vi "Update Lists From BIMS Server.vi"(4 "error IN":errorcluster, 6 "Site":string, 7 "Lookup Table Name":string) -> (0 "error OUT":errorcluster, 3 "recordset data":string[][](array[string]))   [LabVIEW 2010]
uses:
  <vilib>/addons/database/Connection.llb/DB Tools Open Connec (Path).vi
  <vilib>/addons/database/Connection.llb/Conn Execute.vi
  <vilib>/addons/database/Recordset.llb/Rec Destroy - Connection.vi
  <vilib>/addons/database/NI_Database_API.lvlib
panel:
  out "SP Call":string
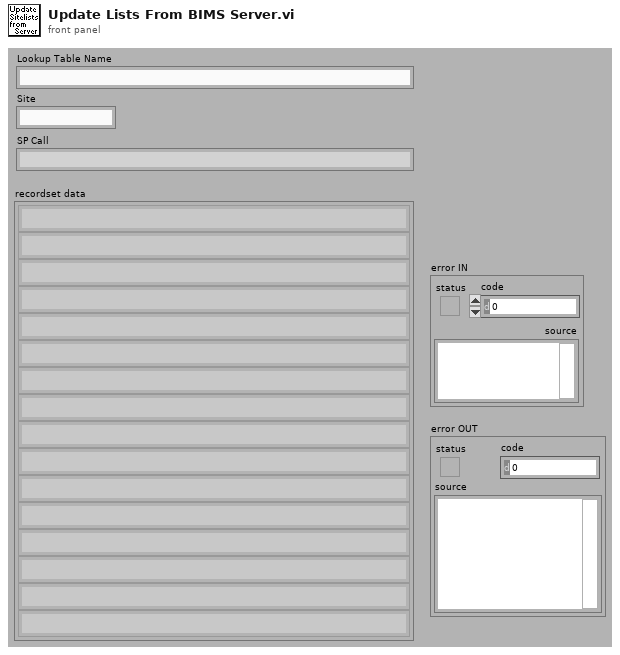
[diagram p1: front panel]
types:
  T1 = typedef "NI_Database_API.lvlib/Conn ObjectReference.ctl" = refnum<k1>
  T2 = typedef "NI_Database_API.lvlib/Rec ObjectReference.ctl" = refnum<k1>
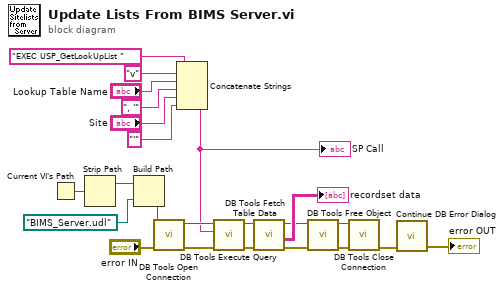
[diagram p0: block diagram]
diagram:
  n1 = Current VI's Path() -> (path=w11:path)
  n2 = Strip Path(path=w11) -> (stripped path=w10:path)  [unwired: 1 out]
  n3 = Build Path(base path=w10, name or relative path=path "BIMS_Server.udl" ("connectString")) -> (appended path=w8:path)
  n4 = call-poly <vilib>:"DB Tools Open Connection.vi"("error in (no error)"="error IN", "connection information"=w8) -> ("error out"=w16:errorcluster, "connection reference"=w14:T1)  [unwired: 3 in, 3 out]
  n5 = Concatenate Strings("EXEC USP_GetLookUpList " ("string"), "v" ("string"), "Lookup Table Name", ", '", "Site", "'") -> (w7:string)
  "SP Call" <- w7
  n6 = call-poly <vilib>:"DB Tools Execute Query.vi"("error in (no error)"=w16, "SQL query"=w7, "connection reference"=w14) -> ("error out"=w17:errorcluster, "recordset reference"=w13:T2)  [unwired: 1 in, 4 out]
  n7 = call <vilib>:"DB Tools Fetch Table Data.vi"("error in (no error)"=w17, "recordset reference"=w13) -> ("error out"=w18:errorcluster, "recordset data"=→"recordset data":string[][], "recordset reference out"=w12:T2)  [unwired: 3 out]
  n8 = call-poly <vilib>:"DB Tools Free Object.vi"("error in (no error)"=w18, "recordset reference"=w12) -> ("error out"=w19:errorcluster, "connection reference"=w15:T1)  [unwired: 8 out]
  n9 = call <vilib>:"DB Tools Close Connection.vi"("error in (no error)"=w19, "connection reference"=w15) -> ("error out"=w21:errorcluster)  [unwired: 5 out]
  n10 = call "Continue DB Error Dialog.vi"("error in (no error)"=w21) -> ("error out"=→"error OUT":errorcluster)  [unwired: 3 in, 2 out]
